vi "数据上传14.vi"(1 "数据数组":string[](array[string]), 4 "产品ID":string) -> ()   [LabVIEW 2013]
uses:
  <vilib>/Utility/error.llb/whitespace.ctl
panel:
  in  "error in (no error)":errorcluster
  out "error out":errorcluster
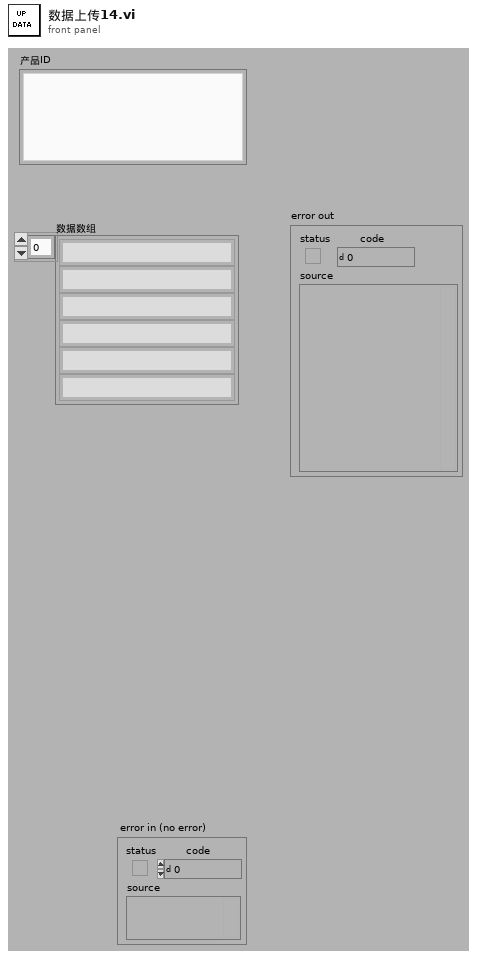
[diagram p1: front panel]
types:
  T1 = typedef "whitespace.ctl" = u16
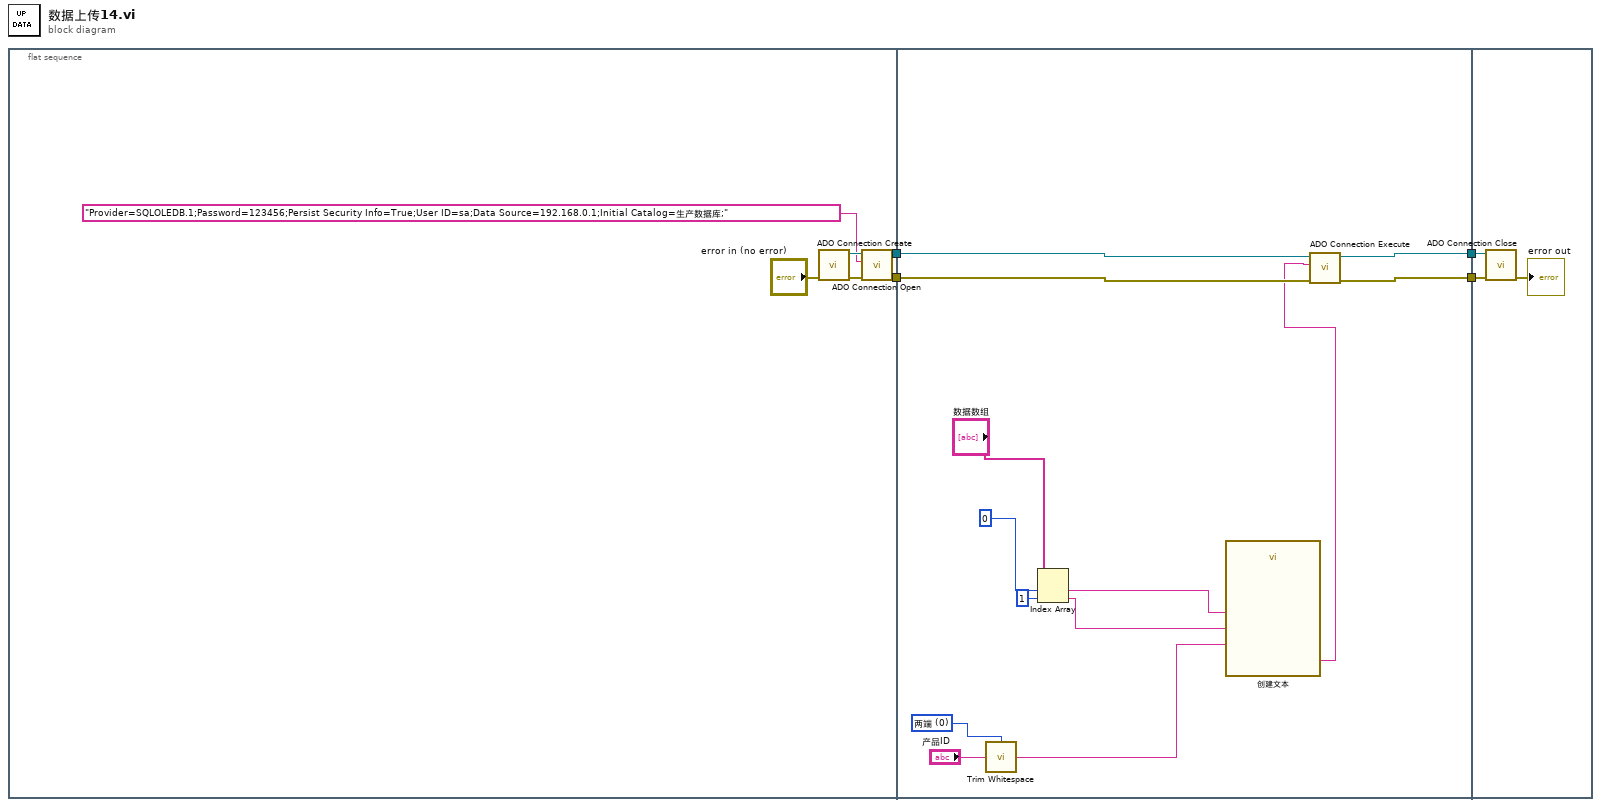
[diagram p0: block diagram]
diagram:
  n1 = flat-sequence {
    tunnel: [w6] -> w4
    tunnel: [w7] -> w3
    tunnel: w4 -> [w23]
    tunnel: w3 -> [w22]
    tunnel: [w18] -> w2
    tunnel: [w17] -> w1
    tunnel: w2 -> [w25]
    tunnel: w1 -> [w24]
    frame #0 {
      n2 = call "ADO Connection Create.vi"("error in (no error)"="error in (no error)") -> ("error out"=w9:errorcluster, "ADODB._Connection Out"=w8:refnum<k7>)  [unwired: 9 out]
      n3 = call "ADO Connection Open.vi"("error in (no error)"=w9, "ConnectionString"="Provider=SQLOLEDB.1;Password=123456;Persist Security Info=True;User ID=sa;Data Source=192.168.0.1;Initial Catalog=生产数据库;" ("字符串 2"), "ADODB._Connection In"=w8) -> ("error out"=w6:errorcluster, "ADODB._Connection Out"=w7:refnum<k7>)  [unwired: 7 out]
    }
    frame #1 {
      w21 = T1 0 items=["两端", "字符串首端", "字符串末端"] ("location (both)")
      n4 = call <vilib>:"Trim Whitespace.vi"("string"="产品ID", "location (both)"=w21) -> ("trimmed string"=w11:string)
      n5 = Index Array(array="数据数组", index #1=0 ("索引"), index #2=1 ("索引")) -> (element #1=w13:string, element #2=w12:string)
      n6 = call "创建文本"("员工ID"=w13, "合格"=w12, "产品ID"=w11) -> ("Result"=w15:string)  [unwired: 11 in, 1 out]
      n7 = call "ADO Connection Execute.vi"("error in (no error)"=w23, "CommandText"=w15, "ADODB._Connection In"=w22) -> ("error out"=w17:errorcluster, "ADODB._Connection Out"=w18:refnum<k7>)  [unwired: 7 out]
    }
    frame #2 {
      n8 = call "ADO Connection Close.vi"("error in (no error)"=w24, "ADODB._Connection In"=w25) -> ("error out"=→"error out":errorcluster)  [unwired: 9 out]
    }
  }
